vi "OpenVISA.vi"(8 "error in (no error)":errorcluster, 11 "ConfocalStage in":refnum<class "ConfocalStage.lvclass">) -> (0 "error out":errorcluster, 3 "ConfocalStage out":refnum<class "ConfocalStage.lvclass">)   [LabVIEW 2012, in "ConfocalStage.lvclass"]
uses:
  ConfocalStage.lvclass
  ConfocalStage.lvclass/ConfocalStage.ctl
  <vilib>/Instr/_visa.llb/VISA Configure Serial Port (Instr).vi
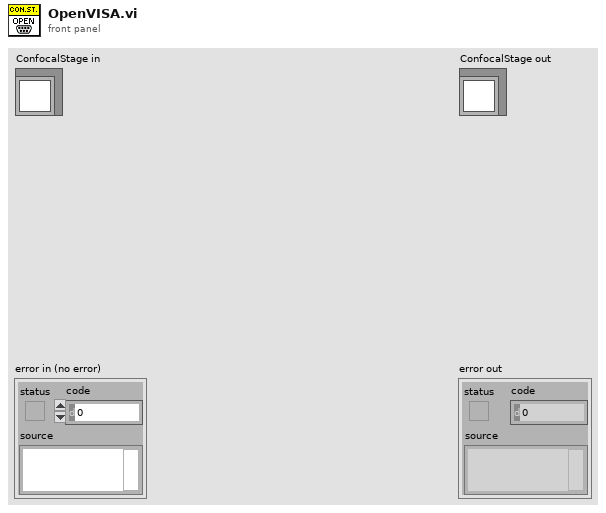
[diagram p1: front panel]
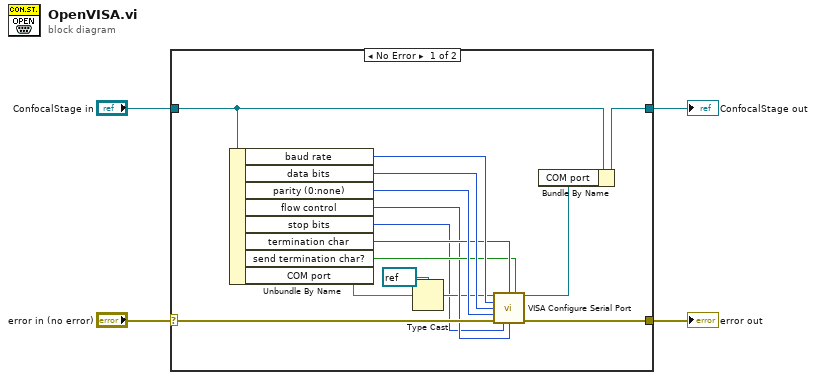
[diagram p0: block diagram]
diagram:
  n1 = case shown="No Error" "error in (no error)" {
    selector: "error in (no error)" -> [w19 w21]
    tunnel: [w18 w21] -> w3
    tunnel: [w10 w20] -> w1
    tunnel: "ConfocalStage in" -> [w11 w20]
    frame No Error {
      n2 = Unbundle By Name(w11) -> ("baud rate"=w17:u32, "data bits"=w16:u16, "parity (0:none)"=w15:enum16{"None", "Odd", "Even", "Mark", "Space"}, "flow control"=w12:u16, "stop bits"=w5:u16, "termination char"=w14:u8, "send termination char?"=w13:bool, "COM port"=w8:string)
      n3 = Type Cast(type=refnum<visa-resource-name> refnum ("VISA resource name"), x=w8) -> (*(type *) &x=w6:refnum<visa-resource-name>)
      n4 = call-poly "VISA Configure Serial Port"("VISA resource name"=w6, "termination char\n(0xA = '\\n' = LF)"=w14, "Enable Termination\nChar (T)"=w13, "baud rate (9600)"=w17, "data bits (8)"=w16, "parity (0:none)"=w15, "error in (no error)"=w19, "stop bits (10: 1 bit)"=w5, "flow control (0:none)"=w12) -> ("VISA resource name out"=w9:refnum<visa-resource-name>, "error out"=w18:errorcluster)  [unwired: 5 in]
      n5 = Bundle By Name(cluster=w11, "COM port"=w9) -> (w10:refnum<class "ConfocalStage.lvclass">)
    }
    frame Error {
    }
  }
  "error out" <- w3
  "ConfocalStage out" <- w1
